vi "File or directory exists.vi"(8 "error in (no error)":errorcluster, 10 "Path":string, 11 "WebDAV in":refnum<class "WebDAV.lvclass">) -> (0 "error out":errorcluster, 1 "Exists?":bool, 2 "Path out (dup)":string, 3 "WebDAV out":refnum<class "WebDAV.lvclass">, 4 "Type":T1)   [LabVIEW 2016, in "RT Management.lvlib" / "WebDAV.lvclass"]
uses:
  WebDAV.lvclass
  C:/GitHub/SystemManagementAndInformation/source/classes/File Transfer Behavior/File Transfer Behavior.lvclass
  File Transfer Behavior/Type.ctl
  WebDAV.lvclass/WebDAV.ctl
  Get Session.vi
  <vilib>/Utility/error.llb/Trim Whitespace.vi
  <vilib>/WebDAVClient/NI_WebDAV.lvlib
  File Transfer Behavior/File Transfer Behavior.lvclass
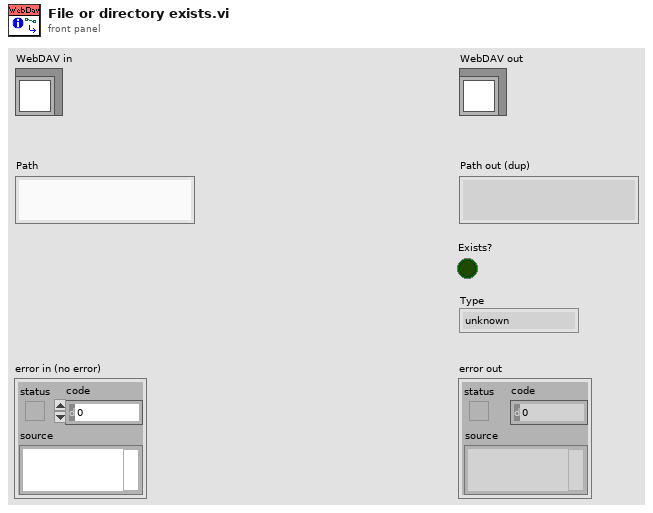
[diagram p1: front panel]
types:
  T1 = typedef "RT Management.lvlib/File Transfer Behavior.lvclass/Type.ctl" = enum16{"unknown", "file", "directory"}
  T2 = typedef "NI_WebDAV.lvlib/SessionHandle.ctl" = refnum<k1>
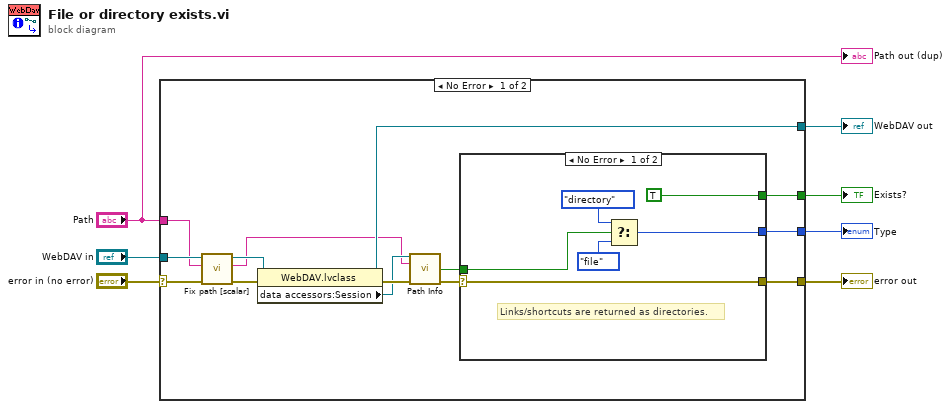
[diagram p0: block diagram]
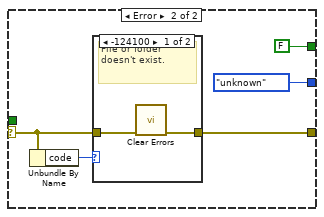
[diagram p2: hidden frame]
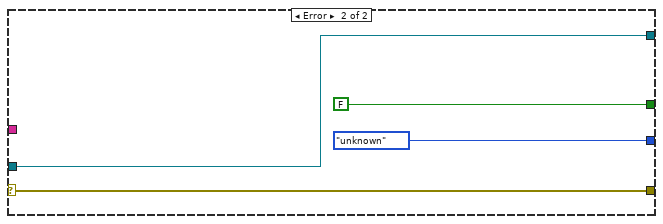
[diagram p4: hidden frame]
diagram:
  n1 = case shown="No Error" "error in (no error)" {
    selector: "error in (no error)" -> [w20 w39]
    tunnel: [w15 w39] -> w6
    tunnel: "WebDAV in" -> [w19 w38]
    tunnel: [w14 w38] -> w4
    tunnel: "Path" -> [w12 _]
    tunnel: [w9 FALSE ("Exists?")] -> w2
    tunnel: [w8 Type."unknown" ("Type")] -> w1
    frame No Error {
      n2 = call "Fix path [scalar].vi"("error in (no error)"=w20, "Path in"=w12, "File Transfer Behavior in"=w19) -> ("error out"=w17:errorcluster, "Path out"=w13:string, "File Transfer Behavior out"=w16:refnum<class "WebDAV.lvclass">)  [unwired: 6 in]
      n3 = property class="WebDAV.lvclass"(reference=w16, error in=w17) -> (reference out=w14:refnum<class "WebDAV.lvclass">, error out=w21:errorcluster, "data accessors:Session"=w18:T2)
      n4 = call <vilib>:"Path Info.vi"("session handle"=w18, "relative uri"=w13, "error in (no error)"=w21) -> ("is directory?"=w10:bool, "error out"=w11:errorcluster)  [unwired: 9 in, 2 out]
      n5 = case shown="No Error" w11 {
        selector: w11 -> [w27 w30]
        tunnel: [w27 w32] -> w15
        tunnel: w10 -> [w26 _]
        tunnel: [TRUE ("Exists?") FALSE ("Exists?")] -> w9
        tunnel: [w25 Type."unknown" ("Type")] -> w8
        frame No Error {
          # "Links/shortcuts are returned as directories."
          n6 = Select(t=Type."directory" ("Type"), s=w26, f=Type."file") -> (s? t:f=w25:T1)
        }
        frame Error {
          n7 = Unbundle By Name(w30) -> ("code"=w31:i32)
          n8 = case shown="-124100" w31 {
            tunnel: [w33 w35] -> w32
            tunnel: w30 -> [w34 w35]
            frame -124100 {
              # "File or folder doesn't exist."
              n9 = call <vilib>:"Clear Errors.vi"("error in (no error)"=w34) -> ("error out"=w33:errorcluster)  [unwired: 5 in, 1 out]
            }
            frame Default {
            }
          }
        }
      }
    }
    frame Error {
    }
  }
  "error out" <- w6
  "WebDAV out" <- w4
  "Exists?" <- w2
  "Type" <- w1
  "Path out (dup)" <- "Path"
